vi "Set Alias.vi"(8 "error in (no error)":errorcluster caption="错误输入（无错误）", 10 "Alias":string, 11 "Item输入":refnum<class "Item.lvclass">) -> (0 "error out":errorcluster caption="错误输出", 3 "Item输出":refnum<class "Item.lvclass">)   [LabVIEW 2013, in "Hierarchy Framework.lvlib" / "Item.lvclass"]
uses:
  Item.lvclass
  Item.lvclass/Item.ctl
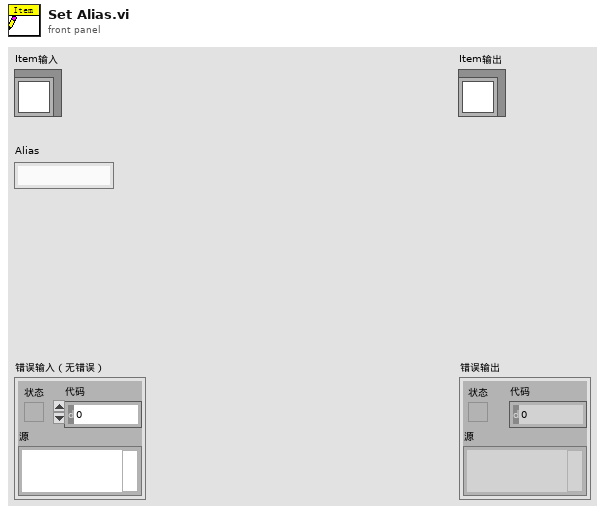
[diagram p1: front panel]
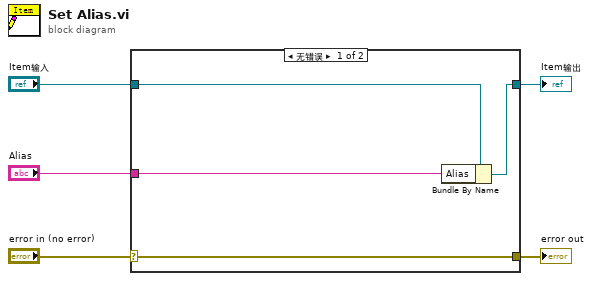
[diagram p0: block diagram]
diagram:
  n1 = case shown="无错误" "error in (no error)" {
    selector: "error in (no error)" -> [w9 w10]
    tunnel: [w9 w10] -> w4
    tunnel: [w7 w11] -> w2
    tunnel: "Item输入" -> [w8 w11]
    tunnel: "Alias" -> [w6 _]
    frame No Error {
      n2 = Bundle By Name(cluster=w8, "Alias"=w6) -> (w7:refnum<class "Item.lvclass">)
    }
    frame Error {
    }
  }
  "error out" <- w4
  "Item输出" <- w2
